vi "Find Net Charge.vi"(8 "error in (no error)":errorcluster, 11 "DFT Path":path) -> (0 "error out":errorcluster, 2 "Net Electrons":i32, 3 "Net Charge":i32)   [LabVIEW 2010]
panel:
  out "Structure Contributed Electrons":i32
  out "#  Used Electrons":i32
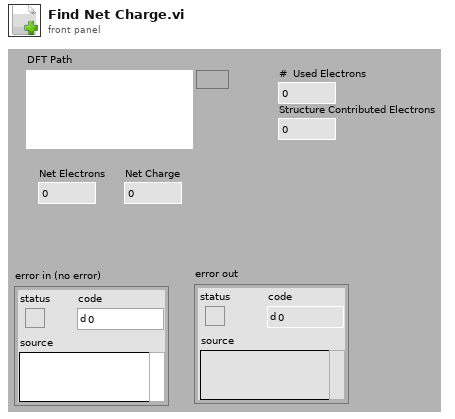
[diagram p1: front panel]
types:
  T1 = cluster{"Structure Name":string, "Lattice vector a":dbl[], "Lattice vector b":dbl[], "Lattice vector c":dbl[], "Atoms Array":cluster{"Atom Name":string, "Positions (Direct)":dbl[][], "Positions (Cartesian)":dbl[][]}[], "# of atoms":i32}
  T2 = cluster{"Atom Name":string, "Positions (Direct)":dbl[][], "Positions (Cartesian)":dbl[][]}[]
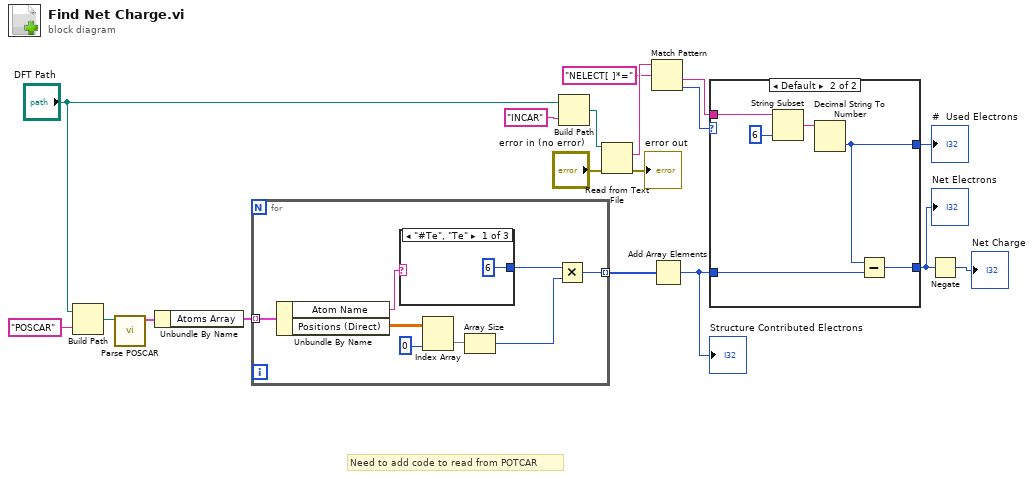
[diagram p0: block diagram]
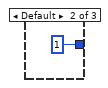
[diagram p3: hidden frame]
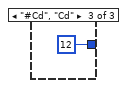
[diagram p4: hidden frame]
diagram:
  # "Need to add code to read from POTCAR"
  n1 = Build Path(base path="DFT Path", name or relative path="POSCAR") -> (appended path=w15:path)
  n2 = call "Parse POSCAR.vi"("POSCAR File"=w15) -> ("Structure"=w16:T1)  [unwired: 7 in, 3 out]
  n3 = Unbundle By Name(w16) -> ("Atoms Array"=w18:T2)
  n4 = for {
    tunnel: w18 -> [w26] mode=indexing
    tunnel: [w21] -> w17 mode=indexing
    n5 = Unbundle By Name(w26) -> ("Atom Name"=w20:string, "Positions (Direct)"=w25:dbl[][])
    n6 = case shown="\"#Te\", \"Te\"" w20 {
      tunnel: [6 ("x") 1 ("x") 12 ("x")] -> w19
      frame "#Te", "Te" {
      }
      frame Default {
      }
      frame "#Cd", "Cd" {
      }
    }
    n7 = Index Array(array=w25, index (col)=0 ("disabled index (col)")) -> (element=w23:dbl[])  [unwired: 1 in]
    n8 = Array Size(array=w23) -> (size(s)=w22:i32)
    n9 = Multiply(x=w19, y=w22) -> (x*y=w21:i32)
  }
  n10 = Build Path(base path="DFT Path", name or relative path="INCAR") -> (appended path=w11:path)
  n11 = Read from Text File(file (use dialog)=w11, error in="error in (no error)") -> (text=w10:string, error out=→"error out":errorcluster)  [unwired: 2 in, 2 out]
  n12 = Match Pattern(string=w10, regular expression="NELECT[ ]*=") -> (after substring=w6:string, offset past match=w7:i32)  [unwired: 1 in, 2 out]
  n13 = Add Array Elements(numeric array=w17) -> (sum=w8:i32)
  "Structure Contributed Electrons" <- w8
  n14 = case shown="Default" w7 {
    tunnel: w6 -> [_ w35]
    tunnel: w8 -> [_ w32]
    tunnel: [_ w31] -> w5
    tunnel: [_ w30] -> w3
    frame -1 {
    }
    frame Default {
      n15 = String Subset(string=w35, length (rest)=6 ("length (rest)")) -> (substring=w33:string)  [unwired: 1 in]
      n16 = Decimal String To Number(string=w33) -> (number=w30:i32)  [unwired: 2 in, 1 out]
      n17 = Subtract(x=w30, y=w32) -> (x-y=w31:i32)
    }
  }
  "Net Electrons" <- w5
  "#  Used Electrons" <- w3
  n18 = Negate(x=w5) -> (-x=→"Net Charge":i32)
